vi "Dispense Schedule.vi"() -> (6 "Dispense Times":dbl[](array[numeric])=[0.0, 3600.0, 7200.0, 10800.0, 14400.0, 18000.0] format="%<%H:%M>t", 7 "Dispense Schedule":dbl[](array[numeric])=[10.72, 10.72, 10.72, 10.72, 10.72, 10.72] format="%.2f", 8 "Flow Rate Schedule":dbl[](array[numeric])=[3.0, 3.0, 3.0, 3.0, 3.0, 3.0] format="%.2f", 9 "Temperature Schedule":dbl[](array[numeric])=[58.0, 58.0, 58.0, 58.0, 58.0, 58.0] format="%.2f")   [LabVIEW 2012]
panel:
  in  "stop":bool
  in  "Flow Rate":dbl[](array[numeric])=[3.0, 3.0, 3.0, 3.0, 3.0, 3.0] format="%.2f"
  in  "Incoming Water Temperature":dbl[](array[numeric])=[58.0, 58.0, 58.0, 58.0, 58.0, 58.0] format="%.2f"
  in  "Dispense Times":dbl[](array[numeric])=[0.0, 3600.0, 7200.0, 10800.0, 14400.0, 18000.0] format="%<%H:%M>t"
  in  "Total Gallons":dbl[](array[numeric])=[10.72, 10.72, 10.72, 10.72, 10.72, 10.72] format="%.2f"
  # "Set Your Desired Dispense Pattern.\nPress \"Complete\" to use default values"
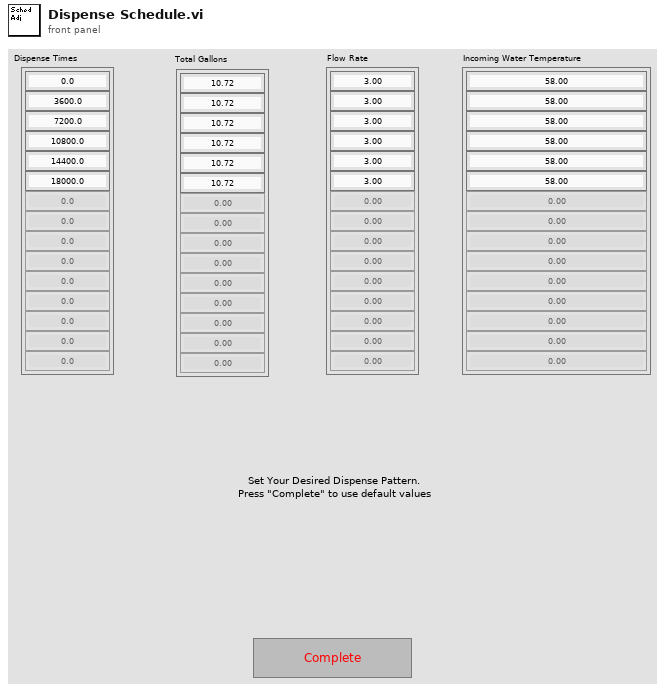
[diagram p1: front panel]
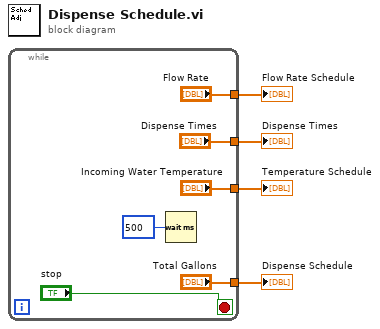
[diagram p0: block diagram]
diagram:
  n1 = while {
    tunnel: ["Dispense Times"] -> w1
    tunnel: ["Total Gallons"] -> w2
    tunnel: ["Incoming Water Temperature"] -> w3
    tunnel: ["Flow Rate"] -> w4
    stop <- "stop" stop-if-true
    n2 = Wait (ms)(milliseconds to wait=u32 500) -> ()  [unwired: 1 out]
  }
  "Dispense Times" <- w1
  "Dispense Schedule" <- w2
  "Temperature Schedule" <- w3
  "Flow Rate Schedule" <- w4
